vi "Polarization_Simulation.vi"() -> ()   [LabVIEW 2018]
panel:
  in  "Drive Zero Level Down":bool
  in  "Thermally Connect Zero Ensemble":bool
  in  "Zero Ensemble Power":dbl=0.05
  in  "Zero Lorentzian Position":dbl=1.0
  in  "Zero Lorentzian Width":dbl=0.05
  in  "Zero Ensemble Area":dbl=0.1
  in  "Zero Level on":bool
  in  "Gaussian Noise SD":dbl
  in  "AFP Efficiency":dbl=0.8
  in  "Timing (ms)":i32=10
  out "XY Graph 3":cluster{dbl[], "rho- out":dbl[]}[](graph)
  in  "AFP Sweep Direction":u16(ring) items=["Positive", "Negative"]
  in  "RF Proportional to Intensity":bool
  in  "File operation":u16(ring) items=["Open existing file", "Create new file", "Replace existing file"]
  out "XY Graph 2":cluster{"Array":dbl[], "Array 2":dbl[]}(graph)
  in  "Sweep AFP Range":bool
  in  "RF Power":dbl=0.1 min=0.0 max=1.0 step=0.01
  in  "Also use RF Range 2":bool
  in  "RF on":bool
  out "XY Graph":cluster{dbl[], "rho+ array out":dbl[]}[](graph)
  in  "Microwave on":bool
  in  "AFP Slider":cluster{i32, i32}(slide)={0, 500} scale=0.0..500.0
  in  "RF Slider 2":cluster{i32, i32}(slide)={0, 4} scale=0.0..500.0
  in  "RF Slider 1":cluster{i32, i32}(slide)={201, 238} scale=0.0..500.0
  in  "Relaxation Rate":dbl min=0.0 max=1.0 step=0.0001
  in  "Microwave Power":dbl=0.05 min=0.0 max=1.0 step=0.001
  in  "Saturation Polarization":dbl=0.45 min=0.0 max=0.99 step=0.01
  in  "Signal Lorentzian Width":dbl=0.005 min=0.0 step=0.001
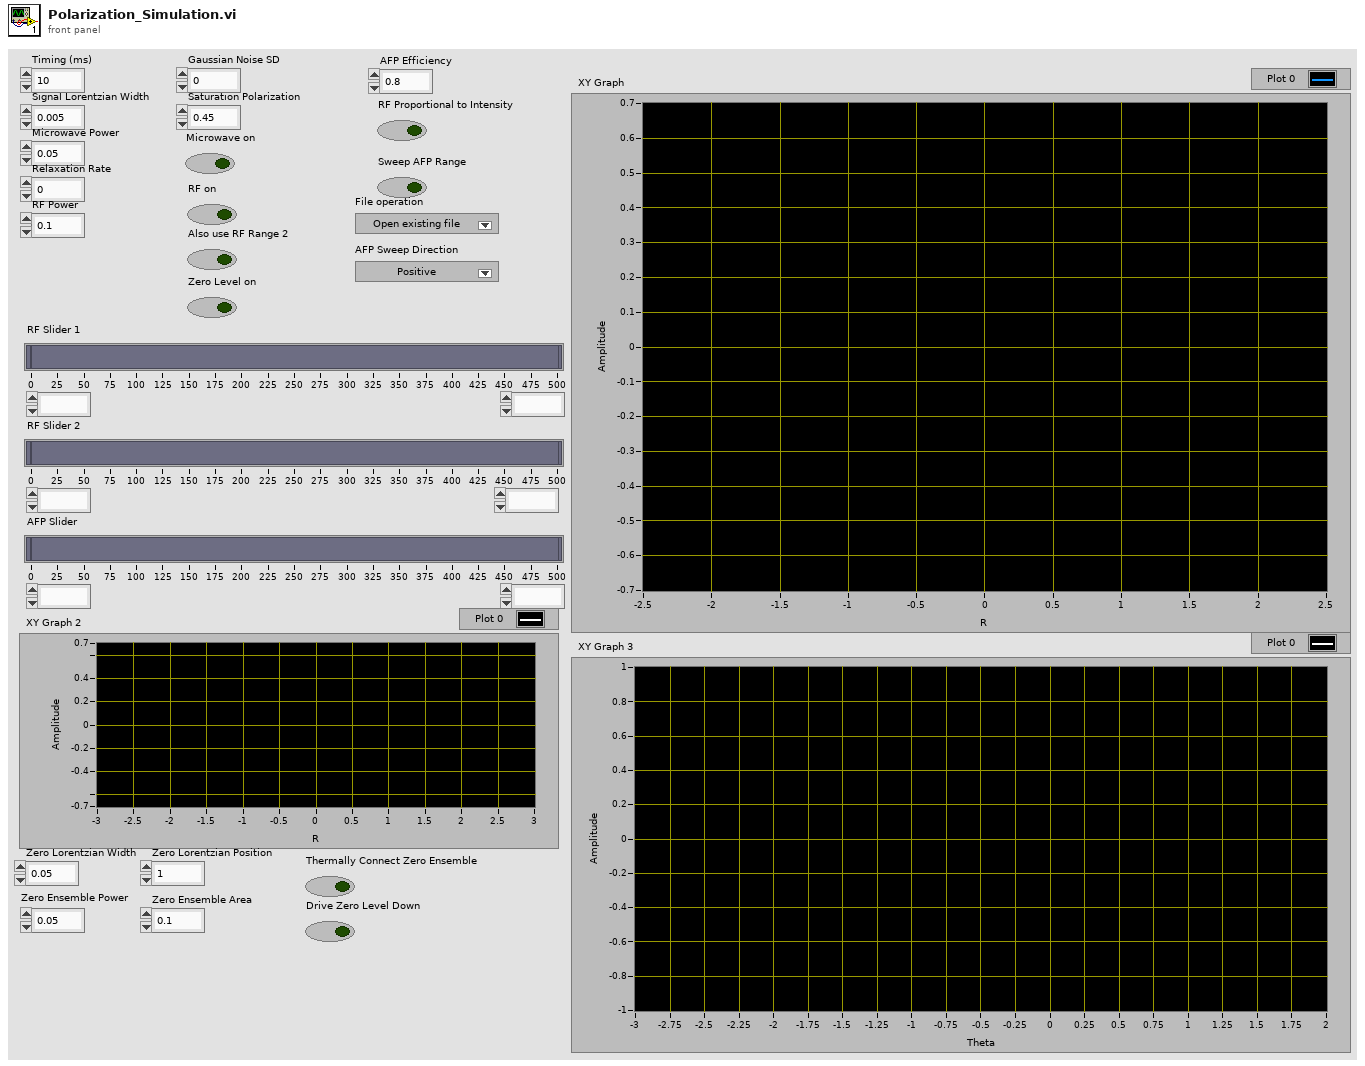
[diagram p1: front panel]
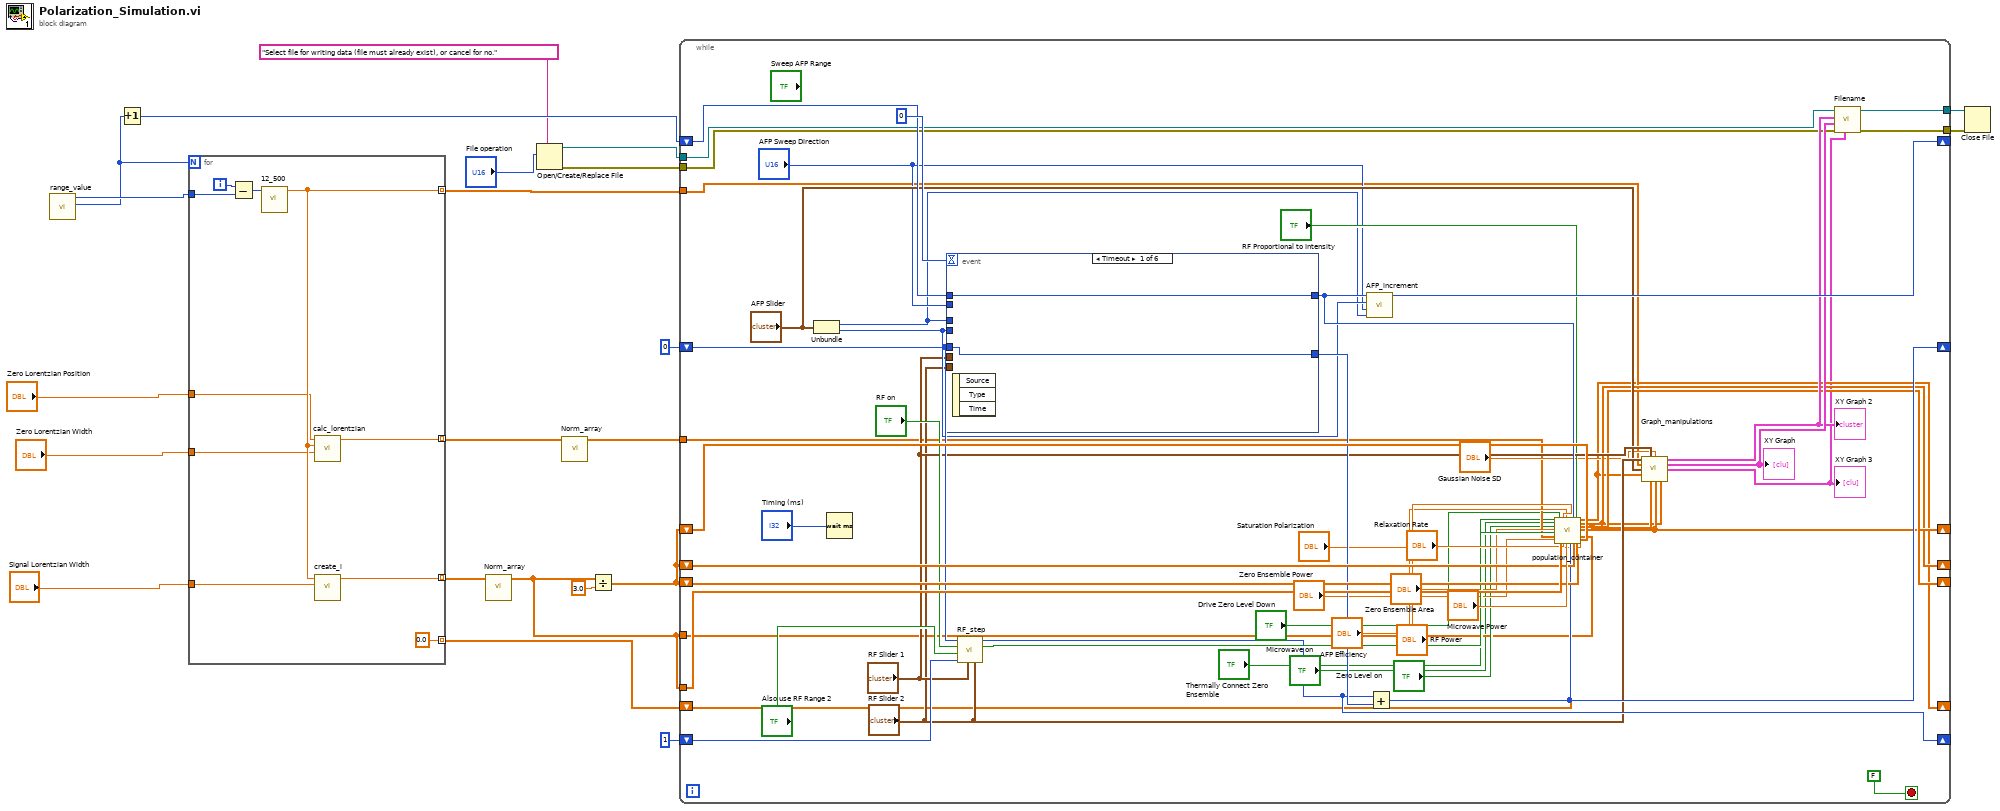
[diagram p0: block diagram]
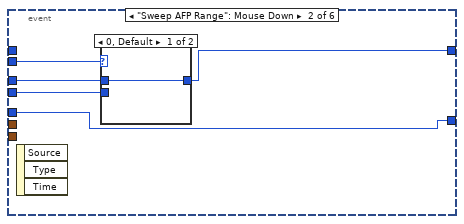
[diagram p2: hidden frame]
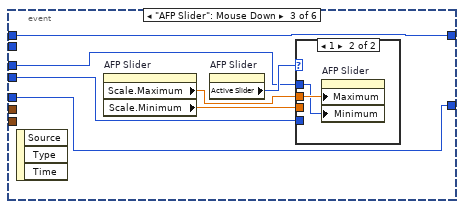
[diagram p4: hidden frame]
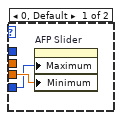
[diagram p5: hidden frame]
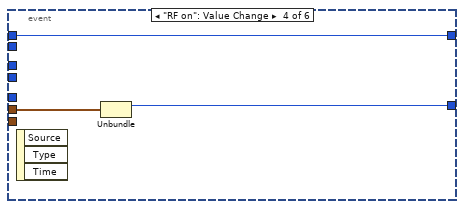
[diagram p6: hidden frame]
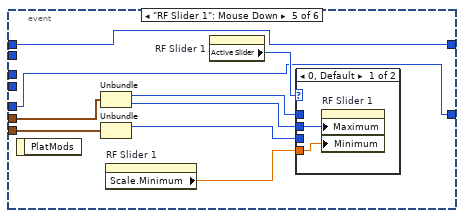
[diagram p7: hidden frame]
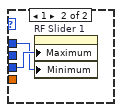
[diagram p8: hidden frame]
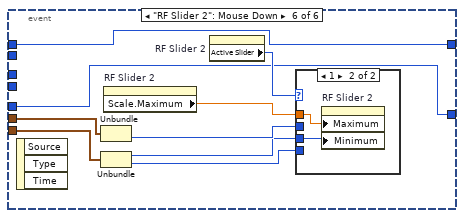
[diagram p9: hidden frame]
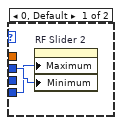
[diagram p10: hidden frame]
diagram:
  n1 = call "range_value.vi"() -> ("NumBins"=w16:i32, "Center"=w22:i32)  [unwired: 10 in]
  n2 = Increment(x=w16) -> (x+1=w15:i32)
  n3 = for {
    N: w16 -> [_]
    tunnel: [w30] -> w20 mode=indexing
    tunnel: w22 -> [w29]
    tunnel: "Signal Lorentzian Width" -> [w28]
    tunnel: [w26] -> w19 mode=indexing
    tunnel: [w27] -> w6 mode=indexing
    tunnel: "Zero Lorentzian Width" -> [w25]
    tunnel: "Zero Lorentzian Position" -> [w24]
    tunnel: [0.0] -> w2 mode=indexing
    i -> [w32]
    n4 = Subtract(x=w32, y=w29) -> (x-y=w31:i32)
    n5 = call "12_500.vi"("Numeric in"=w31) -> ("Numeric out"=w26:dbl)  [unwired: 10 in]
    n6 = call "calc_lorentzian.vi"("Width in"=w25, "x in"=w26, "Position in"=w24) -> ("Value out"=w27:dbl)  [unwired: 8 in]
    n7 = call "create_i.vi"("Lorentzian Width"=w28, "Numeric"=w26) -> ("Numeric 2"=w30:dbl)  [unwired: 9 in]
  }
  n8 = call "Norm_array.vi"("Array"=w20) -> ("Normed Array"=w1:dbl[])  [unwired: 10 in]
  n9 = Open/Create/Replace File(prompt="Select file for writing data (file must already exist), or cancel for no.", operation (0:open)="File operation") -> (refnum out=w12:refnum<file>, error out=w14:errorcluster)  [unwired: 4 in, 1 out]
  n10 = call "Norm_array.vi"("Array"=w6) -> ("Normed Array"=w3:dbl[])  [unwired: 10 in]
  n11 = Divide(x=w1, y=3.0) -> (x/y=w7:dbl[])
  n12 = while {
    tunnel: w1 -> [w83]
    shift-right: [w51] -> _
    shift-left: w7 -> [w80]
    shift-right: [w49] -> _
    shift-left: w7 -> [w78]
    shift-right: [w50] -> _
    shift-left: w7 -> [w79]
    tunnel: w19 -> [w38]
    shift-right: [w70] -> _
    shift-left: 1 -> [w68]
    shift-right: [w72] -> _
    shift-left: 0 -> [w69]
    shift-right: [w66] -> _
    shift-left: w15 -> [w67]
    tunnel: w14 -> [w58]
    tunnel: [w57] -> w13
    tunnel: w12 -> [w56]
    tunnel: [w55] -> w11
    tunnel: w3 -> [w44]
    shift-right: [w37] -> _
    shift-left: w2 -> [w43]
    tunnel: w1 -> [w34]
    stop <- FALSE stop-if-true
    n13 = Unbundle("AFP Slider") -> (w52:i32, w64:i32)
    n14 = Wait (ms)(milliseconds to wait="Timing (ms)") -> ()  [unwired: 1 out]
    n15 = event shown="[0] Timeout" {
      selector: _ -> [_ _ _ _ _ _]
      dyn-events: _ -> [_ _ _ _ _ _]
      timeout: 0 -> [_ _ _ _ _ _]
      tunnel: "RF Slider 2" -> [_ _ _ _ w111 w129]
      tunnel: "RF Slider 1" -> [_ _ _ w107 w112 w128]
      tunnel: [w86 w91 w94 w106 w109 w122] -> w73
      tunnel: w69 -> [w86 w91 w94 _ w109 w122]
      tunnel: [w85 w88 w95 w105 w108 w121] -> w65
      tunnel: w67 -> [w85 _ w95 w105 w108 w121]
      tunnel: w52 -> [_ w87 w97 _ _ _]
      tunnel: w64 -> [_ w89 w96 _ _ _]
      tunnel: "AFP Sweep Direction" -> [_ w90 _ _ _ _]
      event Timeout {
        n16 = event-data() -> ()  [unwired: 1 in, 3 out]
      }
      event "Sweep AFP Range": Mouse Down {
        n17 = event-data() -> ()  [unwired: 1 in, 3 out]
        n18 = case shown="0, Default" w90 {
          tunnel: [w92 w93] -> w88
          tunnel: w89 -> [_ w93]
          tunnel: w87 -> [w92 _]
          frame 0, Default {
          }
          frame 1 {
          }
        }
      }
      event "AFP Slider": Mouse Down {
        n19 = event-data() -> ()  [unwired: 1 in, 3 out]
        n20 = property on="AFP Slider" class="Slide (strict)"() -> ("Scale.Maximum"=w99:dbl, "Scale.Minimum"=w98:dbl)  [unwired: 2 in, 2 out]
        n21 = property on="AFP Slider" class="Slide (strict)"() -> ("Active Slider"=w100:i32)  [unwired: 2 in, 2 out]
        n22 = case shown="1" w100 {
          tunnel: w99 -> [_ w104]
          tunnel: w98 -> [w102 _]
          tunnel: w97 -> [_ w103]
          tunnel: w96 -> [w101 _]
          frame 0, Default {
            n23 = property on="AFP Slider" class="Slide (strict)"("Maximum"=w101, "Minimum"=w102) -> ()  [unwired: 2 in, 2 out]
          }
          frame 1 {
            n24 = property on="AFP Slider" class="Slide (strict)"("Maximum"=w104, "Minimum"=w103) -> ()  [unwired: 2 in, 2 out]
          }
        }
      }
      event "RF on": Value Change {
        n25 = event-data() -> ()  [unwired: 1 in, 3 out]
        n26 = Unbundle(w107) -> (w106:i32)  [unwired: 1 out]
      }
      event "RF Slider 1": Mouse Down {
        n27 = event-data() -> ()  [unwired: 1 in, 1 out]
        n28 = Unbundle(w112) -> (w115:i32, w114:i32)
        n29 = Unbundle(w111) -> (w110:i32)  [unwired: 1 out]
        n30 = property on="RF Slider 1" class="Slide (strict)"() -> ("Scale.Minimum"=w113:dbl)  [unwired: 2 in, 2 out]
        n31 = property on="RF Slider 1" class="Slide (strict)"() -> ("Active Slider"=w116:i32)  [unwired: 2 in, 2 out]
        n32 = case shown="0, Default" w116 {
          tunnel: w110 -> [_ w120]
          tunnel: w115 -> [_ w119]
          tunnel: w114 -> [w118 _]
          tunnel: w113 -> [w117 _]
          frame 0, Default {
            n33 = property on="RF Slider 1" class="Slide (strict)"("Maximum"=w118, "Minimum"=w117) -> ()  [unwired: 2 in, 2 out]
          }
          frame 1 {
            n34 = property on="RF Slider 1" class="Slide (strict)"("Maximum"=w120, "Minimum"=w119) -> ()  [unwired: 2 in, 2 out]
          }
        }
      }
      event "RF Slider 2": Mouse Down {
        n35 = event-data() -> ()  [unwired: 1 in, 3 out]
        n36 = Unbundle(w128) -> (w126:i32)  [unwired: 1 out]
        n37 = Unbundle(w129) -> (w124:i32, w125:i32)
        n38 = property on="RF Slider 2" class="Slide (strict)"() -> ("Scale.Maximum"=w123:dbl)  [unwired: 2 in, 2 out]
        n39 = property on="RF Slider 2" class="Slide (strict)"() -> ("Active Slider"=w127:i32)  [unwired: 2 in, 2 out]
        n40 = case shown="1" w127 {
          tunnel: w126 -> [w131 _]
          tunnel: w125 -> [w130 _]
          tunnel: w124 -> [_ w133]
          tunnel: w123 -> [_ w132]
          frame 0, Default {
            n41 = property on="RF Slider 2" class="Slide (strict)"("Maximum"=w130, "Minimum"=w131) -> ()  [unwired: 2 in, 2 out]
          }
          frame 1 {
            n42 = property on="RF Slider 2" class="Slide (strict)"("Maximum"=w132, "Minimum"=w133) -> ()  [unwired: 2 in, 2 out]
          }
        }
      }
    }
    n43 = call "RF_step.vi"("RF Range 2"="RF Slider 2", "RF Range 1"="RF Slider 1", "RF Step Value"=w68, "2 ranges?"="Also use RF Range 2", "RF on"="RF on", "RF Location"=w69) -> ("RF Indicator"=w74:bool, "RF Location out"=w70:i32)  [unwired: 4 in]
    n44 = call "AFP_increment.vi"("AFP Min"=w52, "Sweep Direction"="AFP Sweep Direction", "AFP Max"=w64, "AFP Target"=w65) -> ("AFP Target Out"=w66:i32)  [unwired: 7 in]
    n45 = Add(x=w70, y=w73) -> (x+y=w72:i32)
    n46 = call "population_container.vi"("Thermally Connect Zero Ensemble"="Thermally Connect Zero Ensemble", "Microwave on"="Microwave on", "Zero Level on"="Zero Level on", "Zero Ensemble Area"="Zero Ensemble Area", "RF Indicator"=w74, "Normed Array 2"=w44, "Zero Ensemble Power"="Zero Ensemble Power", "Drive Zero Level Down"="Drive Zero Level Down", "Normed Array 3"=w83, "RF Power"="RF Power", "Relaxation Rate"="Relaxation Rate", "AFP Efficiency"="AFP Efficiency", "Microwave Power"="Microwave Power", "Numeric 2"=w72, "Array"=w43, "Numeric"=w65, "Array 2"=w78, "RF Proportional to Intensity"="RF Proportional to Intensity", "Array 4"=w80, "Normed Array"=w34, "Array 3"=w79, "Saturation Polarization"="Saturation Polarization") -> ("Zero ensemble out"=w37:dbl[], "rho- out"=w49:dbl[], "rho+ out"=w51:dbl[], "rho0 out"=w50:dbl[])  [unwired: 2 in]
    n47 = call "Graph_manipulations.vi"("RF Slider in"="RF Slider 2", "RF Slider 1"="RF Slider 1", "Gaussian Noise SD"="Gaussian Noise SD", "Array in"=w38, "AFP Slider"="AFP Slider", "Zero ensemble in"=w37, "rho+ in"=w51, "rho0 in"=w50, "rho- in"=w49) -> ("Q Graph"=w59:cluster{"Array":dbl[], "Array 2":dbl[]}, "P Graph and Intensities and RF"=w60:cluster{"Array":dbl[], "Array":dbl[]}[], "Array out"=w36:cluster{dbl[], "Zero ensemble out":dbl[]}[])  [unwired: 4 in]
    "XY Graph" <- w60
    "XY Graph 2" <- w59
    "XY Graph 3" <- w36
    n48 = call "Filename.vi"("Densities and De Boer"=w36, "error in (no error)"=w58, "P Graph and Intensities and RF"=w60, "Q Graph"=w59, "Byte Stream File in"=w56) -> ("error out"=w57:errorcluster, "Byte Stream File out"=w55:refnum<file>)  [unwired: 5 in]
  }
  n49 = Close File(refnum=w11, error in=w13) -> ()  [unwired: 2 out]
